vi "Reset Test.vi"() -> ()   [LabVIEW 2014]
panel:
  out "Waveform Chart":i32(graph)
  out "Numeric":dbl
  in  "Boolean":bool
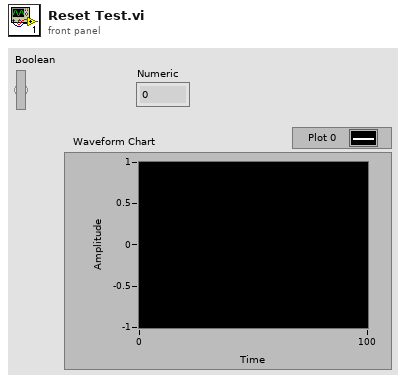
[diagram p1: front panel]
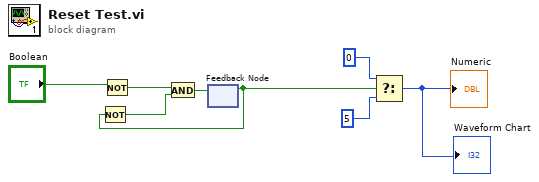
[diagram p0: block diagram]
diagram:
  n1 = Not(x="Boolean") -> (.not. x?=w4:bool)
  n2 = feedback #1() -> (w1:bool)  [unwired: 1 in]
  n3 = Not(x=w1) -> (.not. x?=w3:bool)
  n4 = And(x=w4, y=w3) -> (x .and. y?=w2:bool)
  n5 = feedback-in #1(w2) -> ()
  n6 = Select(t=0, s=w1, f=5) -> (s? t:f=→"Numeric" →"Waveform Chart":i32)
